vi "Loop_ACT_Motors.vi"() -> ()   [LabVIEW 2017, in "Claw.lvlib"]
uses:
  Claw.lvlib
  _SHARE ALL/TypeDef Share All/CLUSTER_PDP_Status.ctl
  _SHARE ALL/TypeDef Share All/CLUSTER_PDP_Faults.ctl
  TypeDef/CLUSTER_Two Motor Output.ctl
  TypeDef/CLUSTER_Two Motor Input.ctl
  Globals/Global_Device_IDs.vi
  <vilib>/Rock Robotics/WPI/RobotDrive/WPI_RobotDriveOpen2MotorWithExistingMotors.vi
  _SHARE ALL/Global Share All/Global_STOP.vi
  Global_SM Write_Data Out.vi
  _SHARE ALL/RoboRio Share All/Systems Share All/System_Monitoring/Global_SEN Write_Data.vi
  Global_ACT Write_Data Out.vi
  _SHARE ALL/RoboRio Share All/Systems Share All/System_Monitoring/System_Status.lvlib
panel:
  out "Claw Output":T1
  in  "PDP Status":T2
  out "Cycle Time (S)":dbl format="%.3g"
  in  "Target Time(ms)":u32=50
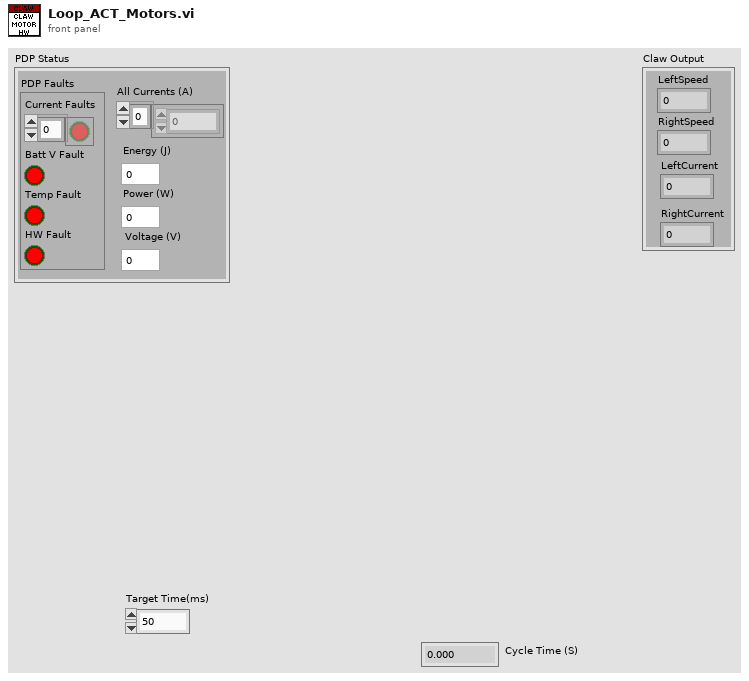
[diagram p1: front panel]
types:
  T1 = typedef "CLUSTER_Two Motor Output.ctl" = cluster{"LeftSpeed":dbl, "RightSpeed":dbl, "LeftCurrent":dbl, "RightCurrent":dbl}
  T2 = typedef "CLUSTER_PDP_Status.ctl" = cluster{"PDP Faults":T3, "All Currents (A)":dbl[], "Energy (J)":dbl, "Power (W)":dbl, "Voltage (V)":dbl}
  T3 = typedef "CLUSTER_PDP_Faults.ctl" = cluster{"Current Faults":bool[], "Batt V Fault":bool, "Temp Fault":bool, "HW Fault":bool}
  T4 = typedef "CLUSTER_Two Motor Input.ctl" = cluster{"LeftSpeed":dbl, "RightSpeed":dbl}
  T5 = typedef "CLUSTER_Claw_Setup.ctl" = cluster{"Left Motor Setup":T6, "Right Motor Setup":T6, "Left Motor PDP":i32, "Right Motor PDP":i32, "Solonoid Setup":T7, "Limit Switch DIO":T9}
  T6 = typedef "CLUSTER_PWM Motor Setup.ctl" = cluster{"Motor ID":u8, "Invert Motor":bool}
  T7 = typedef "CLUSTER_Solonoid_Setup.ctl" = cluster{"Pneumatics Control Module (0)":u8, "Forward Solenoid Channel":T8, "Reverse Solenoid Channel":T8}
  T8 = typedef "WPI_SolenoidChannel.ctl" = enum8{"Solenoid 0", "Solenoid 1", "Solenoid 2", "Solenoid 3", "Solenoid 4", "Solenoid 5", "Solenoid 6", "Solenoid 7", "Invalid"}
  T9 = typedef "FPGA_DIOChannel.ctl" = enum8{"DIO 0", "DIO 1", "DIO 2", "DIO 3", "DIO 4", "DIO 5", "DIO 6", "DIO 7", "DIO 8", "DIO 9", "DIO MXP 0", "DIO MXP 1", "DIO MXP 2", "DIO MXP 3", "DIO MXP 4", "DIO MXP 5", "DIO MXP 6", "DIO MXP 7", "DIO MXP 8", "DIO MXP 9", "DIO MXP 10", "DIO MXP 11", "DIO MXP 12", "DIO MXP 13", "DIO MXP 14", "DIO MXP 15", "SPI Port CS1", "SPI Port CS2", "SPI Port CS3", "SPI Port MISO", "SPI Port MOSI", "Invalid"}
  T10 = typedef "WPI_MotorControlDeviceRef.ctl" = cluster{"DeviceStatus":errorcluster, "Type":T11, "PWM":cluster{"PWM Channel":T12, "DeadBand":T13}, "CAN":cluster{"Device Number":u8, "SetOutput VI Ref":variant, "GetOutput VI Ref":variant, "Enable VI Ref":variant, "Disable VI Ref":variant, "Data":variant}, "Invert":bool, "DIO PWM":cluster{"PWM \"Enable\" Channel":T12, "DIOChannel":T9, "PWM Rate":dbl}}
  T11 = typedef "WPI_MotorControlType.ctl" = enum16{"PWM", "CAN", "DIO PWM"}
  T12 = typedef "FPGA_DIOPWMChannel.ctl" = enum8{"PWM 0", "PWM 1", "PWM 2", "PWM 3", "PWM 4", "PWM 5", "PWM 6", "PWM 7", "PWM 8", "PWM 9", "PWM MXP 0", "PWM MXP 1", "PWM MXP 2", "PWM MXP 3", "PWM MXP 4", "PWM MXP 5", "PWM MXP 6", "PWM MXP 7", "PWM MXP 8", "PWM MXP 9", "Invalid"}
  T13 = typedef "WPI_PWMDeadband.ctl" = cluster{"Name":string, "maxPositivePwm":i32, "minPositivePwm":i32, "centerPwm":i32, "maxNegativePwm":i32, "minNegativePwm":i32, "angularRange":u16}
  T14 = typedef "WPI_RobotDriveDevRef.ctl" = cluster{"DevStatus":errorcluster, "Motors[]":T10[], "Square Inputs":bool, "Max Output":dbl}
  T15 = cluster{"Left Motor PDP":i32, "Right Motor PDP":i32, "RobotDriveDevRef":T14, "Claw Output":T1, "Claw Input":T4, "Target Time(ms)":u32, "Current Time":timestamp, "Previous Time":timestamp, "Cycle Time (S)":dbl, "PDP Status":T2}
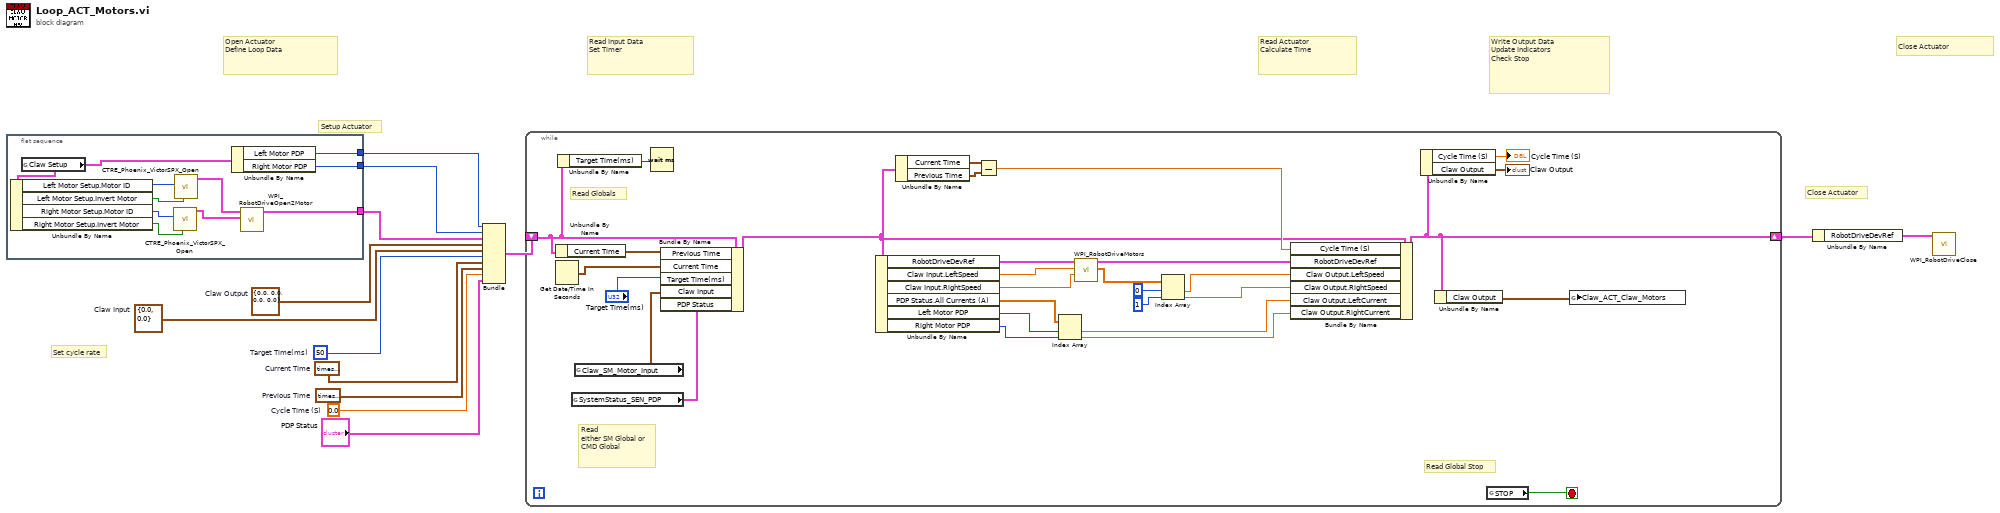
[diagram p0: block diagram]
diagram:
  w5 = T1 {"LeftSpeed"=0.0, "RightSpeed"=0.0, "LeftCurrent"=0.0, "RightCurrent"=0.0}  # Claw Output
  w6 = T4 {"LeftSpeed"=0.0, "RightSpeed"=0.0}  # Claw Input
  w8 = 0.0  # Cycle Time (S)
  w13 = timestamp(0 s since 1904-01-01)  # Previous Time
  w12 = timestamp(0 s since 1904-01-01)  # Current Time
  w11 = u32 50  # Target Time(ms)
  # "Close Actuator"
  # "Write Output Data\nUpdate Indicators\nCheck Stop"
  # "Read Actuator\nCalculate Time"
  # "Read Input Data\nSet Timer"
  # "Open Actuator\nDefine Loop Data"
  # "Set cycle rate"
  # "Close Actuator"
  # "Setup Actuator"
  n1 = flat-sequence {
    tunnel: [w23] -> w7
    tunnel: [w21] -> w2
    tunnel: [w20] -> w1
    frame #0 {
      n2 = global read "Global_Device_IDs.vi" "Claw Setup"() -> (w22:T5)
      n3 = Unbundle By Name(w22) -> ("Left Motor Setup.Motor ID"=w18:u8, "Left Motor Setup.Invert Motor"=w19:bool, "Right Motor Setup.Motor ID"=w17:u8, "Right Motor Setup.Invert Motor"=w16:bool)
      n4 = call "CTRE_Phoenix_VictorSPX_Open.vi"("Invert"=w16, "Device Number"=w17) -> ("CAN Talon SRX Ref"=w15:T10)  [unwired: 8 in, 1 out]
      n5 = call "CTRE_Phoenix_VictorSPX_Open.vi"("Invert"=w19, "Device Number"=w18) -> ("CAN Talon SRX Ref"=w14:T10)  [unwired: 8 in, 1 out]
      n6 = Unbundle By Name(w22) -> ("Left Motor PDP"=w21:i32, "Right Motor PDP"=w20:i32)
      n7 = call-poly <vilib>:"WPI_RobotDriveOpen2Motor.vi"("Right Motor Dev Ref"=w15, "Left Motor Dev Ref"=w14) -> ("RobotDriveDevRef"=w23:T14)  [unwired: 8 in, 1 out]
    }
  }
  n8 = Bundle("Left Motor PDP"=w2, "Right Motor PDP"=w1, "RobotDriveDevRef"=w7, "Claw Output"=w5, "Claw Input"=w6, "Target Time(ms)"=w11, "Current Time"=w12, "Previous Time"=w13, "Cycle Time (S)"=w8, "PDP Status"="PDP Status") -> (w10:T15)  [unwired: 1 in]
  n9 = while {
    shift-right: [w45] -> w9
    shift-left: w10 -> [w47]
    stop <- w53 stop-if-true
    # "Read\neither SM Global or CMD Global"
    # "Read Globals"
    # "Read Global Stop"
    n10 = Unbundle By Name(w47) -> ("Current Time"=w51:timestamp)
    n11 = Get Date/Time In Seconds() -> (seconds since 1Jan1904=w52:timestamp)
    n12 = Unbundle By Name(w47) -> ("Target Time(ms)"=w46:u32)
    n13 = global read "Global_SEN Write_Data.vi" "SystemStatus_SEN_PDP"() -> (w30:T2)
    n14 = global read "Global_SM Write_Data Out.vi" "Claw_SM_Motor_Input"() -> (w41:T4)
    n15 = Wait (ms)(milliseconds to wait=w46) -> ()  [unwired: 1 out]
    n16 = Bundle By Name(cluster=w47, "Previous Time"=w51, "Current Time"=w52, "Target Time(ms)"="Target Time(ms)", "Claw Input"=w41, "PDP Status"=w30) -> (w42:T15)
    n17 = Unbundle By Name(w42) -> ("RobotDriveDevRef"=w32:T14, "Claw Input.LeftSpeed"=w39:dbl, "Claw Input.RightSpeed"=w38:dbl, "PDP Status.All Currents (A)"=w29:dbl[], "Left Motor PDP"=w28:i32, "Right Motor PDP"=w27:i32)
    n18 = Unbundle By Name(w42) -> ("Current Time"=w50:timestamp, "Previous Time"=w49:timestamp)
    n19 = Subtract(x=w50, y=w49) -> (x-y=w43:dbl)
    n20 = Index Array(array=w29, index #1=w28, index #2=w27) -> (element #1=w26:dbl, element #2=w25:dbl)
    n21 = call <vilib>:"WPI_RobotDriveMotors.vi"("RightSpeed"=w38, "LeftSpeed"=w39, "RobotDriveDevRef"=w32) -> ("Motor Values"=w37:dbl[], "RobotDriveDevRef"=w31:T14)  [unwired: 6 in, 1 out]
    n22 = Index Array(array=w37, index #1=0 ("index"), index #2=1 ("index")) -> (element #1=w34:dbl, element #2=w33:dbl)
    n23 = Bundle By Name(cluster=w42, "Cycle Time (S)"=w43, "RobotDriveDevRef"=w31, "Claw Output.LeftSpeed"=w34, "Claw Output.RightSpeed"=w33, "Claw Output.LeftCurrent"=w26, "Claw Output.RightCurrent"=w25) -> (w45:T15)
    n24 = Unbundle By Name(w45) -> ("Cycle Time (S)"=→"Cycle Time (S)":dbl, "Claw Output"=→"Claw Output":T1)
    n25 = Unbundle By Name(w45) -> ("Claw Output"=w40:T1)
    n26 = global read "Global_STOP.vi" "STOP"() -> (w53:bool)
    n27 = global write "Global_ACT Write_Data Out.vi" "Claw_ACT_Claw_Motors"(w40) -> ()
  }
  n28 = Unbundle By Name(w9) -> ("RobotDriveDevRef"=w4:T14)
  n29 = call <vilib>:"WPI_RobotDriveClose.vi"("RobotDriveDevRef"=w4) -> ()  [unwired: 10 in, 1 out]
